vi "stateView.vi"(10 "UserEvents in":refnum<class "UserEvents.lvclass">) -> ()   [LabVIEW 2015, in "M1M3SSSTViews.lvlib"]
uses:
  M1M3SSSTViews.lvlib
  UserEvents/UserEvents.lvclass
  Typedefs/StateSelector.ctl
  UserEvents/UserEvents.lvclass/UserEvents.ctl
  Typedefs/M1M3SSSTypedefs.lvlib
panel:
  out "State:":T1
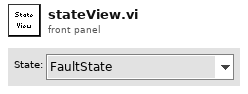
[diagram p1: front panel]
types:
  T1 = typedef "M1M3SSSTypedefs.lvlib/StateSelector.ctl" = enum16{"FaultState", "OffState", "RampingUpPressurePState", "RampingUpPressureSTState", "StandbyState", "StoppedState", "WaitingForSettledPState", "WaitingForSettledSTState"}
  T2 = typedef "M1M3SSSTypedefs.lvlib/PubDataEvents.ctl" = cluster{"State":refnum<user-event>, "ErrorCode":refnum<user-event>, "OutputData":refnum<user-event>, "InputData":refnum<user-event>, "ControllerData":refnum<user-event>, "TestStatus":refnum<user-event>, "LogPath":refnum<user-event>, "StiffnessData":refnum<user-event>, "PreconditioningCycle":refnum<user-event>}
  T3 = cluster{"Event Registration Refnum":refnum<event-registration>}
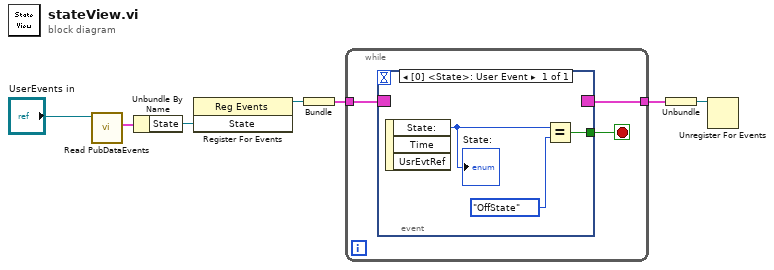
[diagram p0: block diagram]
diagram:
  n1 = call "Read PubDataEvents.vi"("UserEvents in"="UserEvents in") -> ("PubDataEvents"=w5:T2)  [unwired: 9 in, 1 out]
  n2 = Unbundle By Name(w5) -> ("State"=w6:refnum<user-event>)
  n3 = register-events(w6) -> (reference out=w7:refnum<event-registration>)  [unwired: 2 in, 1 out]
  n4 = Bundle("Event Registration Refnum"=w7) -> (w4:T3)  [unwired: 1 in]
  n5 = while {
    tunnel: w4 -> [w10]
    tunnel: [w9] -> w3
    stop <- w8 stop-if-true
    n6 = event shown="[0] <State>: User Event" {
      selector: w10 -> [_]
      dyn-events: [_] -> w9
      timeout: _ -> [_]
      tunnel: [w12] -> w8
      event User Event {
        n7 = event-data() -> ("State:"=w11:T1)  [unwired: 1 in, 2 out]
        "State:" <- w11
        n8 = Equal?(x=w11, y=StateSelector."OffState") -> (x = y?=w12:bool)
      }
    }
  }
  n9 = Unbundle(w3) -> ("Event Registration Refnum"=w2:refnum<event-registration>)
  n10 = Unregister For Events(event registration refnum=w2) -> ()  [unwired: 1 in, 1 out]
